vi "Reshape Map.vi"(11 "Maze (0: Empty, -1: Enemy. >0: Teammate":i32[][](array[numeric])) -> (2 "SelfID":i32, 3 "Map":i32[](array[numeric]))   [LabVIEW 2014, in "Formics.lvclass"]
uses:
  Formics.lvclass
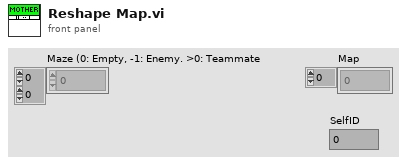
[diagram p1: front panel]
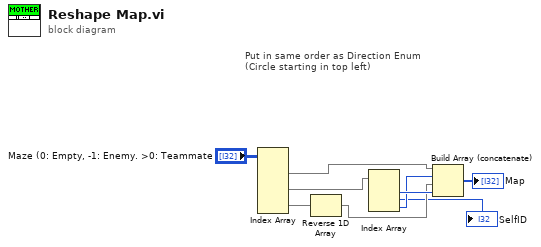
[diagram p0: block diagram]
diagram:
  # "Put in same order as Direction Enum\n(Circle starting in top left)"
  n1 = Index Array(array="Maze (0: Empty, -1: Enemy. >0: Teammate") -> (element #1=w5:i32[], element #2=w4:i32[], element #3=w3:i32[])  [unwired: 6 in]
  n2 = Reverse 1D Array(array=w3) -> (reversed array=w7:i32[])
  n3 = Index Array(array=w4) -> (element #1=w8:i32, element #2=→"SelfID":i32, element #3=w6:i32)  [unwired: 3 in]
  n4 = Build Array (concatenate)(w5, w6, w7, w8) -> (→"Map":i32[])
